vi "Get OOB Server Address.vi"() -> (2 "Boolean":bool, 3 "String":string)   [LabVIEW 2025]
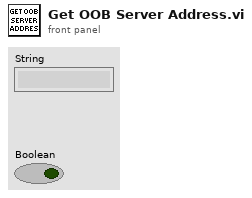
[diagram p1: front panel]
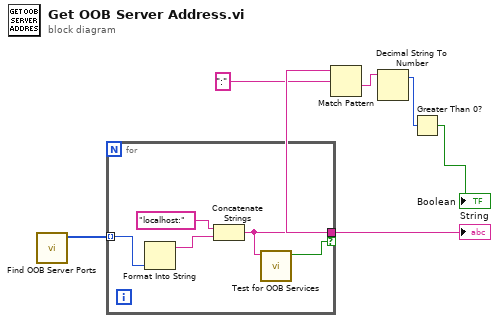
[diagram p0: block diagram]
diagram:
  n1 = call "Find OOB Server Ports.vi"() -> ("Ports"=w1:u16[])  [unwired: 11 in]
  n2 = for {
    tunnel: [w9] -> w3 if=w7
    tunnel: w1 -> [w8] mode=indexing
    n3 = Format Into String(w8) -> (resulting string=w11:string)  [unwired: 3 in, 1 out]
    n4 = Concatenate Strings("localhost:" ("string"), w11) -> (w9:string)
    n5 = call "Test for OOB Services.vi"("address"=w9) -> ("Found OOB Server"=w7:bool)  [unwired: 9 in, 1 out]
  }
  "String" <- w3
  n6 = Match Pattern(string=w3, regular expression=":") -> (after substring=w4:string)  [unwired: 1 in, 3 out]
  n7 = Decimal String To Number(string=w4) -> (offset past number=w5:i32)  [unwired: 2 in, 1 out]
  n8 = Greater Than 0?(x=w5) -> (x > 0?=→"Boolean":bool)
